vi "CRD Timing Diagram.vi"() -> ()   [LabVIEW 2012]
uses:
  <vilib>/measure/NI_MABase.lvlib
panel:
  out "yag":waveform(dbl)[](graph)
  out "diode":waveform(dbl)(graph)
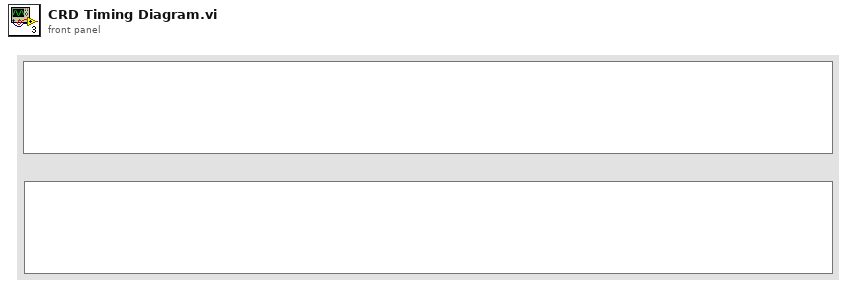
[diagram p1: front panel]
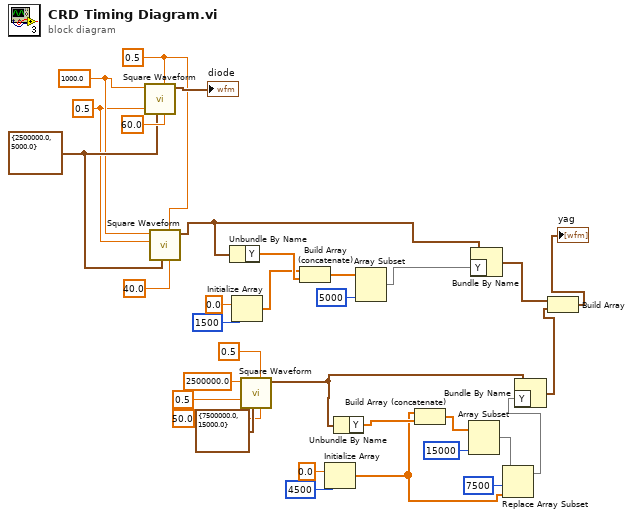
[diagram p0: block diagram]
diagram:
  w19 = 0.5 ("offset")
  w31 = cluster{"Fs":dbl, "#s":dbl} {"Fs"=2500000.0, "#s"=5000.0} ("sampling info")
  w20 = 0.5 ("amplitude")
  w21 = 1000.0 ("frequency")
  n1 = call <vilib>:"Square Waveform.vi"("duty cycle (%)"=60.0, "offset"=w19, "sampling info"=w31, "amplitude"=w20, "frequency"=w21) -> ("signal out"=→"diode":waveform(dbl))  [unwired: 5 in, 1 out]
  n2 = call <vilib>:"Square Waveform.vi"("duty cycle (%)"=40.0, "offset"=w19, "sampling info"=w31, "amplitude"=w20, "frequency"=w21) -> ("signal out"=w22:waveform(dbl))  [unwired: 5 in, 1 out]
  n3 = Unbundle By Name(w22) -> ("Y"=w27:dbl[])
  n4 = Initialize Array(0.0 ("element"), 1500 ("dimension size")) -> (w26:dbl[])
  n5 = call <vilib>:"Square Waveform.vi"("duty cycle (%)"=50.0, "offset"=0.5, "sampling info"=cluster{"Fs":dbl, "#s":dbl} {"Fs"=7500000.0, "#s"=15000.0}, "amplitude"=0.5, "frequency"=2500000.0) -> ("signal out"=w10:waveform(dbl))  [unwired: 5 in, 1 out]
  n6 = Build Array (concatenate)(w26, w27) -> (w25:dbl[])
  n7 = Initialize Array(0.0 ("element"), 4500 ("dimension size")) -> (w7:dbl[])
  n8 = Unbundle By Name(w10) -> ("Y"=w11:dbl[])
  n9 = Array Subset(array=w25, length=5000) -> (w23:dbl[])  [unwired: 1 in]
  n10 = Build Array (concatenate)(w7, w11) -> (w6:dbl[])
  n11 = Array Subset(array=w6, length=15000) -> (w5:dbl[])  [unwired: 1 in]
  n12 = Bundle By Name(cluster=w22, "Y"=w23) -> (w3:waveform(dbl))
  n13 = Replace Array Subset(array=w5, new element=w7, index=7500) -> (w4:dbl[])
  n14 = Bundle By Name(cluster=w10, "Y"=w4) -> (w2:waveform(dbl))
  n15 = Build Array(w3, w2) -> (→"yag":waveform(dbl)[])
